vi "String 2 StringArray.vi"(0 "String":string, 1 "Delimiter (\",\")":string) -> (2 "Substrings":string[](array[string]))   [LabVIEW 2013, in "CS++Utilities.lvlib"]
doc: "This VI converts a <b>String</b> of <b>Delimiter</b> separated substrings into an array of substrings."
uses:
  CS++Utilities.lvlib
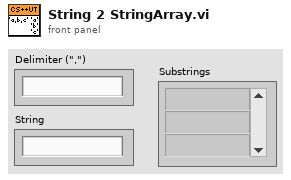
[diagram p1: front panel]
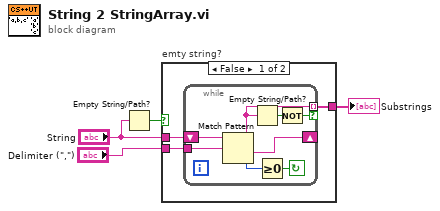
[diagram p0: block diagram]
diagram:
  n1 = Empty String/Path?(string/path="String") -> (empty?=w1:bool)
  n2 = case "emty string?" shown="False" w1 {
    tunnel: "Delimiter (\",\")" -> [w7 _]
    tunnel: [w6 _] -> w3
    tunnel: "String" -> [w5 _]
    frame False {
      n3 = while {
        shift-right: [w14] -> _
        shift-left: w5 -> [w15]
        tunnel: [w10] -> w6 mode=indexing if=w9
        tunnel: w7 -> [w8]
        stop <- w12 continue-if-true
        n4 = Match Pattern(string=w15, regular expression=w8) -> (before substring=w10:string, after substring=w14:string, offset past match=w13:i32)  [unwired: 1 in, 1 out]
        n5 = Empty String/Path?(string/path=w10) -> (empty?=w11:bool)
        n6 = Greater Or Equal To 0?(x=w13) -> (x >= 0?=w12:bool)
        n7 = Not(x=w11) -> (.not. x?=w9:bool)
      }
    }
    frame True {
    }
  }
  "Substrings" <- w3
